vi "Read Float.vi"(8 "error in (no error)":errorcluster, 11 "VISA resource name In":refnum<visa-resource-name>) -> (0 "error out":errorcluster, 2 "float":dbl, 3 "VISA resource name out":refnum<visa-resource-name>)   [LabVIEW 2009, in "Newport 1830-C.lvlib"]
doc: "Reads a float from the output buffer of the instrument."
uses:
  Newport 1830-C.lvlib
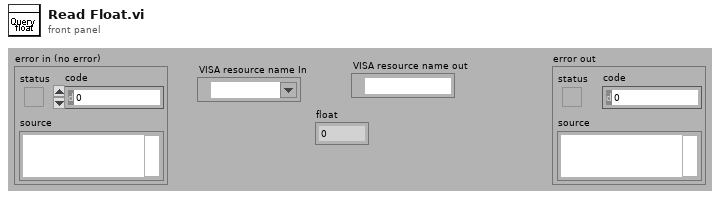
[diagram p1: front panel]
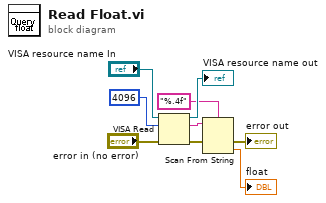
[diagram p0: block diagram]
diagram:
  n1 = VISA Read(VISA resource name="VISA resource name In", byte count=u32 4096, error in (no error)="error in (no error)") -> (VISA resource name out=→"VISA resource name out":refnum<visa-resource-name>, read buffer=w4:string, error out=w5:errorcluster)  [unwired: 1 out]
  n2 = Scan From String(format string="%.4f", input string=w4, error in=w5) -> (error out=→"error out":errorcluster, output 1=→"float":dbl)  [unwired: 2 in, 2 out]
